vi "Islem.vi"(8 "Wait time(s)":i32, 9 "Ýþlem":string="Update Durum", 11 "queue":refnum<queue>) -> ()   [LabVIEW 2021]
panel:
  out "output cluster":T1
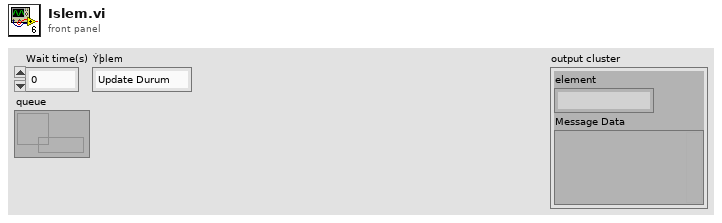
[diagram p1: front panel]
types:
  T1 = cluster{"element":string, "Message Data":variant}
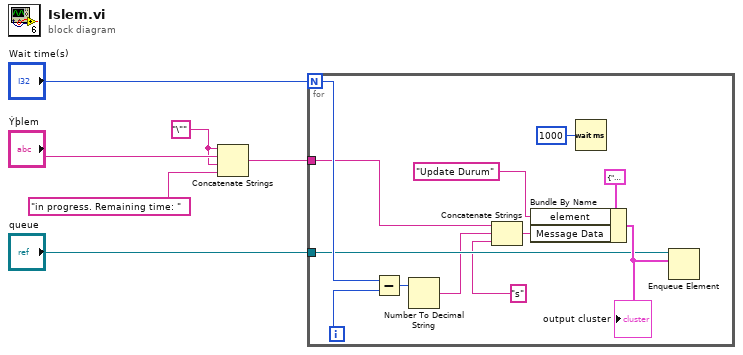
[diagram p0: block diagram]
diagram:
  w3 = "\"" ("string")
  n1 = Concatenate Strings(w3, "Ýþlem", w3, "in progress. Remaining time: " ("string")) -> (w1:string)
  n2 = for {
    N: "Wait time(s)" -> [w14]
    tunnel: "queue" -> [w12]
    tunnel: w1 -> [w11]
    i -> [w13]
    n3 = Subtract(x=w14, y=w13) -> (x-y=w10:i32)
    n4 = Number To Decimal String(number=w10) -> (decimal integer string=w9:string)  [unwired: 1 in]
    n5 = Concatenate Strings(w11, w9, "s" ("string")) -> (w7:string)
    n6 = Bundle By Name(cluster=T1 {"element"="", "Message Data"=variant}, "element"="Update Durum", "Message Data"=w7) -> (w17:T1)
    "output cluster" <- w17
    n7 = Wait (ms)(milliseconds to wait=u32 1000) -> ()  [unwired: 1 out]
    n8 = Enqueue Element(queue=w12, element=w17) -> ()  [unwired: 2 in, 3 out]
  }
